vi "Clamp_MAXMain Function.vi"(0 "Refnum in":T3, 2 "Clamp Settings":T4, 3 "ROI":T5, 5 "error in (no error)":errorcluster, 8 "Process In":u16(ring)) -> (7 "Line Coordinates":T1(array[cluster]) {"?"."Y" format="%.2f"; "?"."X" format="%.2f"; "?"."Y" format="%.2f"; "?"."X" format="%.2f"}, 9 "appended array":cluster{"X":sgl, "Y":sgl}[](array[cluster]), 11 "Perpendicular Lines":T1(array[cluster]), 13 "Points":cluster{"X":sgl, "Y":sgl}[](array[cluster]), 14 "Refnum out":T3, 16 "Distance":sgl, 17 "Edge Coordinates":cluster{"X":sgl, "Y":sgl}[](array[cluster]) {"Y" format="%.2f"; "X" format="%.2f"}, 19 "error out":errorcluster)   [LabVIEW 2015]
uses:
  <vilib>/vision/Image Controls.llb/IMAQ Image.ctl
  <vilib>/vision/NI_Vision_Development_Module.lvlib
panel:
  out "Coordinate System (duplicate)":T2 {"Measurement System"."Axis Reference" items=["Direct", "Indirect"]; "Measurement System"."Angle (deg)" format="%.2f"; "Measurement System"."Origin"."Y" format="%.2f"; "Measurement System"."Origin"."X" format="%.2f"; "Reference System"."Axis Reference" items=["Direct", "Indirect"]; "Reference System"."Angle (deg)" format="%.2f"; "Reference System"."Origin"."Y" format="%.2f"; "Reference System"."Origin"."X" format="%.2f"}
  # "Start Point"
  # "End Point"
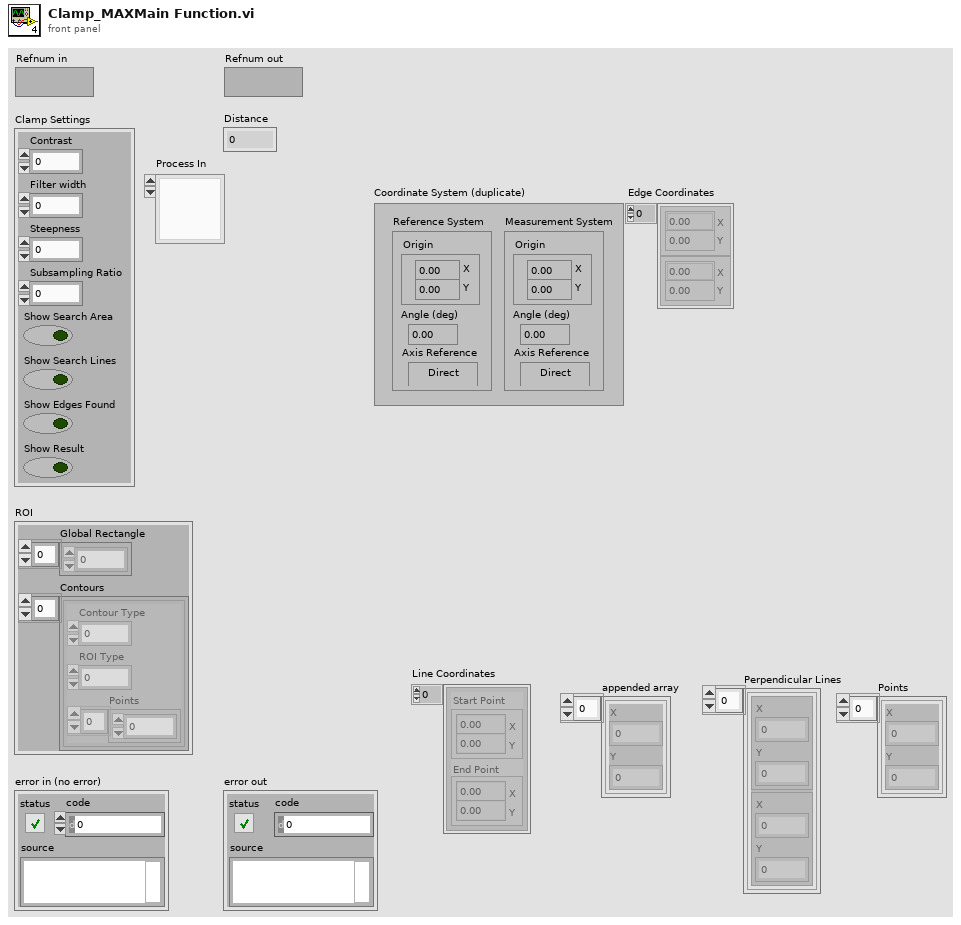
[diagram p1: front panel]
types:
  T1 = cluster{cluster{"X":sgl, "Y":sgl}, cluster{"X":sgl, "Y":sgl}}[]
  T2 = typedef "IMAQ Coordinate System" = cluster{"Reference System":cluster{"Origin":cluster{"X":sgl, "Y":sgl}, "Angle (deg)":sgl, "Axis Reference":u32}, "Measurement System":cluster{"Origin":cluster{"X":sgl, "Y":sgl}, "Angle (deg)":sgl, "Axis Reference":u32}}
  T3 = typedef "IMAQ Image.ctl" = refnum<image>
  T4 = cluster{"Contrast":i32, "Filter width":i32, "Steepness":i32, "Subsampling Ratio":u32, "Show Search Area":bool, "Show Search Lines":bool, "Show Edges Found":bool, "Show Result":bool}
  T5 = cluster{"Global Rectangle":i32[], "Contours":cluster{"Contour Type":u32, "ROI Type":u32, "Points":i32[]}[]}
  T6 = typedef "IMAQ Rectangle" = cluster{"Left":i32, "Top":i32, "Right":i32, "Bottom":i32, "Rotation":dbl}
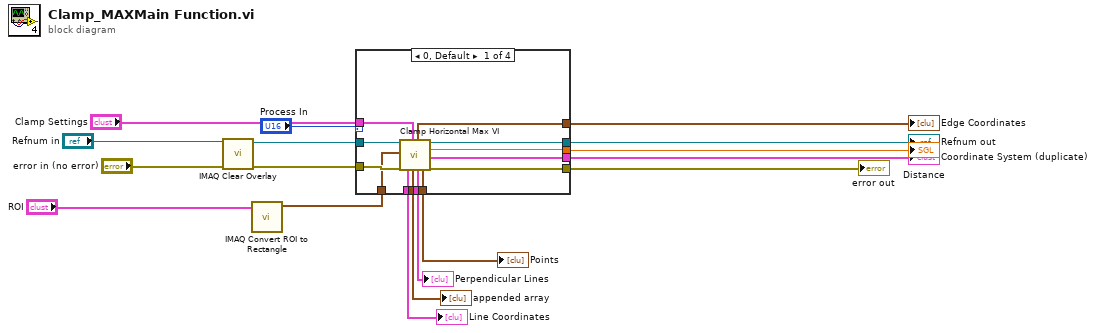
[diagram p0: block diagram]
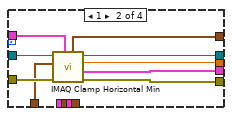
[diagram p2: hidden frame]
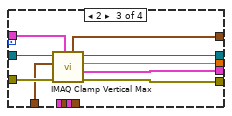
[diagram p3: hidden frame]
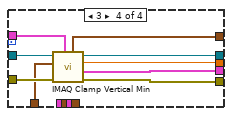
[diagram p4: hidden frame]
diagram:
  n1 = call "IMAQ Clear Overlay"("error in (no error)"="error in (no error)", "Image"="Refnum in") -> ("error out"=w7:errorcluster, "Image Out"=w8:T3)  [unwired: 8 in]
  n2 = call "IMAQ Convert ROI to Rectangle"("ROI Descriptor"="ROI") -> ("Rectangle"=w5:T6)  [unwired: 8 in, 1 out]
  n3 = case shown="0, Default" "Process In" {
    tunnel: w7 -> [w30 w39 w48 w57]
    tunnel: w8 -> [w29 w38 w47 w56]
    tunnel: [w28 w37 w46 w55] -> w17
    tunnel: "Clamp Settings" -> [w22 w36 w45 w54]
    tunnel: [w27 w35 w44 w53] -> w15
    tunnel: [w26 w34 w43 w52] -> w13
    tunnel: [w25 w33 w42 w51] -> w11
    tunnel: [w24 w32 w41 w50] -> w10
    tunnel: w5 -> [w23 w31 w40 w49]
    tunnel: [w21 _ _ _] -> w4
    tunnel: [w20 _ _ _] -> w3
    tunnel: [w19 _ _ _] -> w2
    tunnel: [w18 _ _ _] -> w1
    frame 0, Default {
      n4 = call "Clamp Horizontal Max VI.vi"("Image"=w29, "Rectangle"=w23, "error in (no error)"=w30, "Settings"=w22) -> ("Line Coordinates"=w21:T1, "appended array"=w20:cluster{"X":sgl, "Y":sgl}[], "Edge Coordinates"=w24:cluster{"X":sgl, "Y":sgl}[], "Perpendicular Lines"=w19:T1, "Points"=w18:cluster{"X":sgl, "Y":sgl}[], "Image Out"=w26:T3, "Distance"=w28:sgl, "Coordinate System (duplicate)"=w25:T2, "error out"=w27:errorcluster)  [unwired: 7 in]
    }
    frame 1 {
      n5 = call "IMAQ Clamp Horizontal Min"("Settings"=w36, "error in (no error)"=w39, "Rectangle"=w31, "Image"=w38) -> ("error out"=w35:errorcluster, "Coordinate System (duplicate)"=w33:T2, "Distance"=w37:sgl, "Image Out"=w34:T3, "Edge Coordinates"=w32:cluster{"X":sgl, "Y":sgl}[])  [unwired: 3 in]
    }
    frame 2 {
      n6 = call "IMAQ Clamp Vertical Max"("Settings"=w45, "error in (no error)"=w48, "Rectangle"=w40, "Image"=w47) -> ("error out"=w44:errorcluster, "Coordinate System (duplicate)"=w42:T2, "Distance"=w46:sgl, "Image Out"=w43:T3, "Edge Coordinates"=w41:cluster{"X":sgl, "Y":sgl}[])  [unwired: 3 in]
    }
    frame 3 {
      n7 = call "IMAQ Clamp Vertical Min"("Settings"=w54, "error in (no error)"=w57, "Rectangle"=w49, "Image"=w56) -> ("error out"=w53:errorcluster, "Coordinate System (duplicate)"=w51:T2, "Distance"=w55:sgl, "Image Out"=w52:T3, "Edge Coordinates"=w50:cluster{"X":sgl, "Y":sgl}[])  [unwired: 3 in]
    }
  }
  "Distance" <- w17
  "error out" <- w15
  "Refnum out" <- w13
  "Coordinate System (duplicate)" <- w11
  "Edge Coordinates" <- w10
  "Line Coordinates" <- w4
  "appended array" <- w3
  "Perpendicular Lines" <- w2
  "Points" <- w1
